vi "SocialDoor.vi"(9 "Override":bool, 10 "Interaction time":u32, 11 "STOP":bool) -> (2 "Time spent":dbl)   [LabVIEW 2021]
uses:
  <vilib>/Platform/TimedLoop/XDataNode/timing_clust.ctl
  <vilib>/Platform/TimedLoop/XDataNode/nitl_modes.ctl
  <vilib>/Platform/TimedLoop/XDataNode/wakeup.ctl
  <vilib>/DAQmx/write.llb/DAQmx Write (Digital Bool 1Line 1Point).vi
  <vilib>/DAQmx/create/channels.llb/DAQmx Create Channel (DO-Digital Output).vi
  <vilib>/DAQmx/miscellaneous.llb/DAQmx Fill In Error Info.vi
  Global_BeamBreaks.vi
  GlobalSTATE.vi
  <vilib>/platform/TimedLoop/XDataNode/XDataNode.xnode
  <vilib>/Platform/TimedLoop/XDataNode/XDNodeRunTimeDep.lvlib
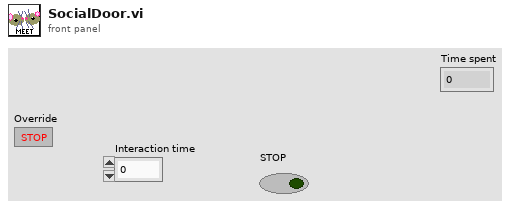
[diagram p1: front panel]
types:
  T1 = typedef "XDNodeRunTimeDep.lvlib/timing_clust.ctl" = cluster{"Expected End [f-1]":u64, "Actual End [f-1]":u64, "Finished Late? [f-1]":bool, "Expected End [i-1]":u64, "Actual End [i-1]":u64, "Finished Late? [i-1]":bool, "Expected Start [i]":u64, "Actual Start [i]":u64, "Expected Start [f]":u64, "Actual Start [f]":u64, "Source Name":string, "Structure Name":string, "Period":i64, "Deadline":i64, "Offset":i64, "Start":i64, "Priority":i32, "Timeout":i32, "Mode":T2, "Wakeup Reason":T3, "Error":errorcluster, "Source Type":string, "Secondary Source Type":string, "Global End Time":u64, "Global Start Time":u64, "Frame Duration":u64, "Iteration Duration":u64, "Assigned CPU":i32, "I/O Scan Engine Mode":u32}
  T2 = typedef "XDNodeRunTimeDep.lvlib/nitl_modes.ctl" = enum32{"No Change", "Process missed periods, maintain original phase", "Discard missed periods, maintain original phase", "Process missed periods, ignore original phase", "Discard missed periods, ignore original phase"}
  T3 = typedef "XDNodeRunTimeDep.lvlib/wakeup.ctl" = enum32{"Normal", "Aborted", "Asynchronous wakeup", "Timing source error", "Timed loop error", "Timeout"}
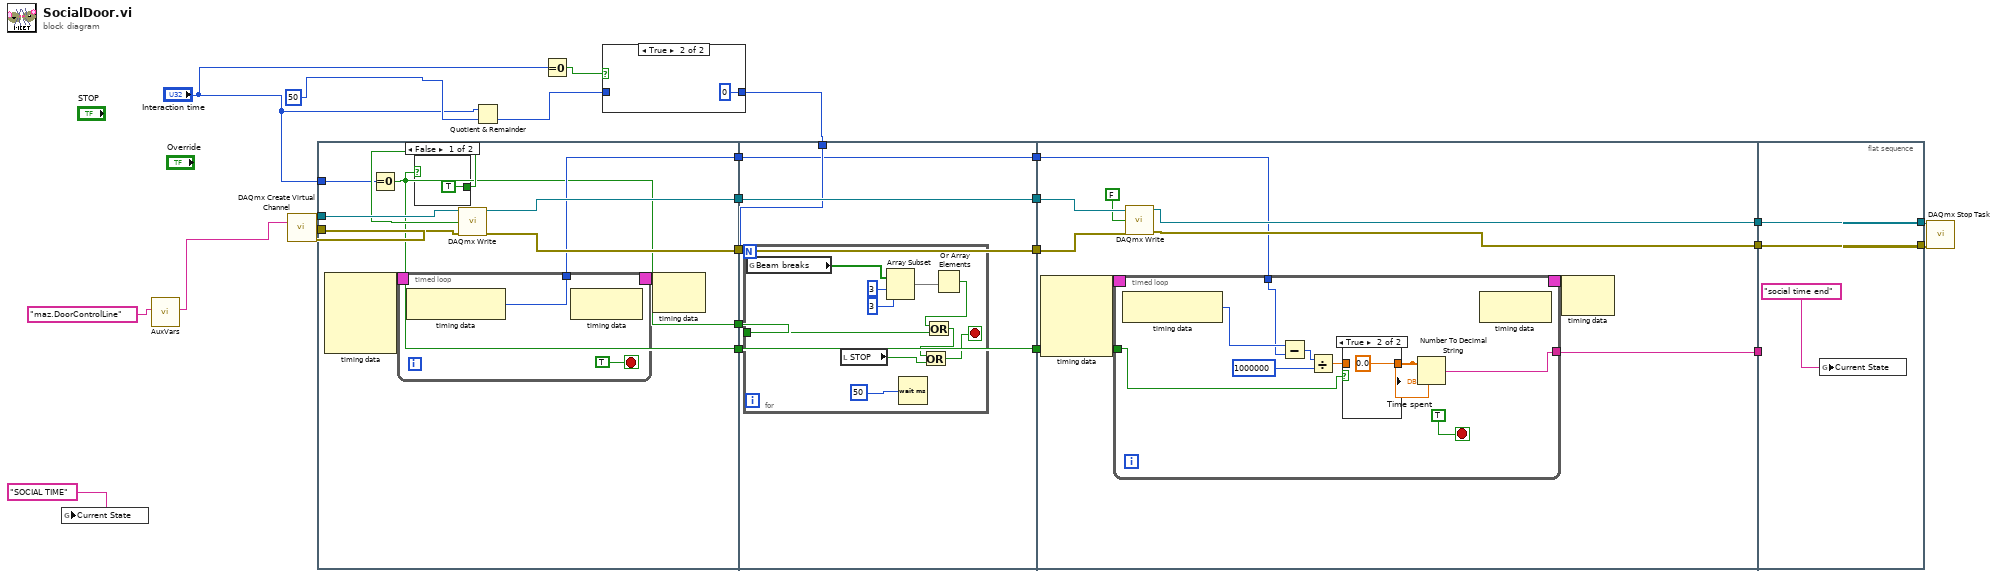
[diagram p0: block diagram]
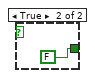
[diagram p3: hidden frame]
diagram:
  n1 = global write "GlobalSTATE.vi" "Current State"("SOCIAL TIME" ("Current State")) -> ()
  n2 = call "AuxVars.vi"("key"="maz.DoorControlLine") -> ("value"=w2:string)  [unwired: 9 in, 1 out]
  n3 = call-poly <vilib>:"DAQmx Create Virtual Channel.vi"("lines"=w2) -> ("task out"=w24:refnum<k21>, "error out"=w21:errorcluster)  [unwired: 13 in]
  n4 = flat-sequence {
    tunnel: w24 -> [w34]
    tunnel: [w33] -> w22
    tunnel: w21 -> [w32]
    tunnel: [w31] -> w19
    tunnel: [w27] -> w13
    tunnel: "Interaction time" -> [w26]
    tunnel: [w25] -> w11
    tunnel: [w25] -> w4
    tunnel: [w49] -> w23
    tunnel: w22 -> [w49]
    tunnel: [w48] -> w20
    tunnel: w19 -> [w48]
    tunnel: w8 -> [w47]
    tunnel: [w46] -> w14
    tunnel: w13 -> [w46]
    tunnel: w11 -> [w45]
    tunnel: [w44] -> w5
    tunnel: w4 -> [w44]
    tunnel: w23 -> [w69]
    tunnel: w20 -> [w68]
    tunnel: [w67] -> w16
    tunnel: [w66] -> w15
    tunnel: w14 -> [w62]
    tunnel: [w61] -> w12
    tunnel: w5 -> [w60]
    tunnel: [w87] -> w17
    tunnel: [w88] -> w18
    tunnel: w16 -> [w88]
    tunnel: w15 -> [w87]
    tunnel: w12 -> [_]
    frame #0 {
      n5 = node-c288() -> (w29:T1)  [unwired: 4 in]
      n6 = Equal To 0?(x=w26) -> (x = 0?=w25:bool)
      n7 = timed-loop {
        timing: w29 -> [_]
        timing-out: [_] -> w28
        tunnel: [w37] -> w27
        stop <- TRUE stop-if-true
        n8 = node-c288() -> (w37:i64)  [unwired: 1 in]
        n9 = node-c288() -> ()  [unwired: 1 in, 1 out]
      }
      n10 = case shown="False" w25 {
        tunnel: [TRUE ("data") FALSE ("data")] -> w30
        frame False {
        }
        frame True {
        }
      }
      n11 = call-poly <vilib>:"DAQmx Write.vi"("task/channels in"=w34, "data"=w30, "error in"=w32) -> ("task out"=w33:refnum<k21>, "error out"=w31:errorcluster)  [unwired: 10 in, 1 out]
      n12 = node-c288(w28) -> ()  [unwired: 1 out]
    }
    frame #1 {
      n13 = for {
        N: w47 -> [_]
        tunnel: w45 -> [w58]
        stop <- w55 stop-if-true
        n14 = global read "Global_BeamBreaks.vi" "Beam breaks"() -> (w52:bool[])
        n15 = local read "STOP"() -> (w57:bool)
        n16 = Array Subset(array=w52, index=3, length=3) -> (w51:bool[])
        n17 = Wait (ms)(milliseconds to wait=u32 50) -> ()  [unwired: 1 out]
        n18 = Or Array Elements(Boolean array=w51) -> (logical OR=w50:bool)
        n19 = Or(x=w50, y=w58) -> (x .or. y?=w56:bool)
        n20 = Or(x=w56, y=w57) -> (x .or. y?=w55:bool)
      }
    }
    frame #2 {
      n21 = node-c288() -> (w64:T1)  [unwired: 4 in]
      n22 = timed-loop {
        timing: w64 -> [_]
        timing-out: [_] -> w63
        tunnel: w62 -> [w76]
        tunnel: [w74] -> w61
        tunnel: w60 -> [w70]
        stop <- TRUE stop-if-true
        n23 = node-c288() -> (w77:i64)  [unwired: 1 in]
        n24 = Subtract(x=w77, y=w76) -> (x-y=w75:i64)
        n25 = Divide(x=w75, y=i64 1000000) -> (x/y=w72:dbl)
        n26 = case shown="True" w70 {
          tunnel: w72 -> [w79 _]
          tunnel: [w79 0.0] -> w71
          frame False {
          }
          frame True {
          }
        }
        "Time spent" <- w71
        n27 = Number To Decimal String(number=w71) -> (decimal integer string=w74:string)  [unwired: 1 in]
        n28 = node-c288() -> ()  [unwired: 1 in, 1 out]
      }
      n29 = call-poly <vilib>:"DAQmx Write.vi"("task/channels in"=w69, "data"=FALSE, "error in"=w68) -> ("task out"=w67:refnum<k21>, "error out"=w66:errorcluster)  [unwired: 10 in, 1 out]
      n30 = node-c288(w63) -> ()  [unwired: 1 out]
    }
    frame #3 {
      n31 = global write "GlobalSTATE.vi" "Current State"("social time end" ("string")) -> ()
    }
  }
  n32 = Quotient & Remainder(x="Interaction time", y=u32 50) -> (floor(x/y)=w9:u32)  [unwired: 1 out]
  n33 = Equal To 0?(x="Interaction time") -> (x = 0?=w7:bool)
  n34 = case shown="True" w7 {
    tunnel: w9 -> [w89 _]
    tunnel: [w89 u32 0] -> w8
    frame False {
    }
    frame True {
    }
  }
  n35 = call <vilib>:"DAQmx Stop Task.vi"("task/channels in"=w18, "error in"=w17) -> ()  [unwired: 12 in, 2 out]
